vi "FA_ConvertToDeviceConfigData.vi"(8 "Error In":errorcluster, 11 "XML String":string) -> (0 "Error Out":errorcluster, 3 "DeviceConfig":T1)   [LabVIEW 2013, in "FA_NativeTypes.lvlib"]
doc: "Converts XML text describing a device configuration to a LabVIEW cluster"
uses:
  FA_NativeTypes.lvlib
  FA_DeviceConfig.ctl
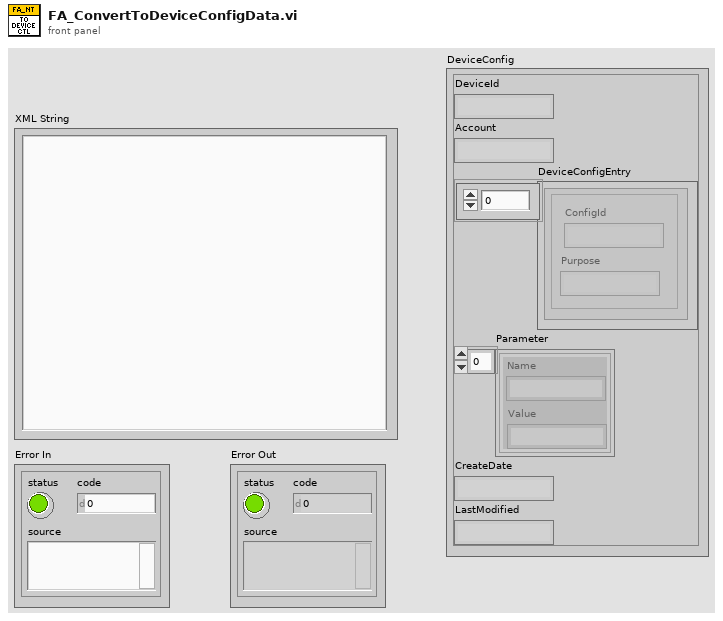
[diagram p1: front panel]
types:
  T1 = typedef "FA_NativeTypes.lvlib/FA_DeviceConfig.ctl" = cluster{"DeviceId":string, "Account":string, "DeviceConfigEntry":cluster{"ConfigId":string, "Purpose":string}[], "Parameter":cluster{"Name":string, "Value":string}[], "CreateDate":string, "LastModified":string}
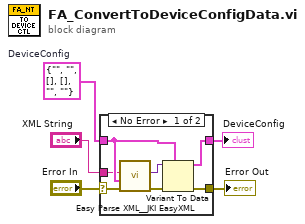
[diagram p0: block diagram]
diagram:
  w3 = T1 {"DeviceId"="", "Account"="", "DeviceConfigEntry"=[], "Parameter"=[], "CreateDate"="", "LastModified"=""}  # DeviceConfig
  n1 = case shown="No Error" "Error In" {
    selector: "Error In" -> [w12 w14]
    tunnel: [w7 w14] -> w4
    tunnel: w3 -> [w9 w13]
    tunnel: [w8 w13] -> w1
    tunnel: "XML String" -> [w6 _]
    frame No Error {
      n2 = call <vilib>:"Easy Parse XML__JKI EasyXML.vi"("error in (no error)"=w12, "LabVIEW Data (Type)"=w9, "XML String"=w6) -> ("error out"=w11:errorcluster, "LabVIEW Data"=w10:variant)  [unwired: 7 in]
      n3 = Variant To Data(error in=w11, type=w9, Variant=w10) -> (data=w8:T1, error out=w7:errorcluster)
    }
    frame Error {
    }
  }
  "Error Out" <- w4
  "DeviceConfig" <- w1
